vi "Sound sample.vi"() -> ()   [LabVIEW 2016]
uses:
  <vilib>/sound2/lvsound2.llb/Sound Data Format.ctl
  <vilib>/sound2/lvsound2.llb/Sound File Info (path).vi
panel:
  out "sound format":T1={"sample rate (S/s)"=22050.0, "number of channels"=2, "bits per sample"=16}
  out "Waveform Graph":waveform(dbl)(graph)
  in  "Sound  Input":path=path "C:/Users/exception/Desktop/MISC/Public Enemy - Harder Than You Think (HQ).mp3"
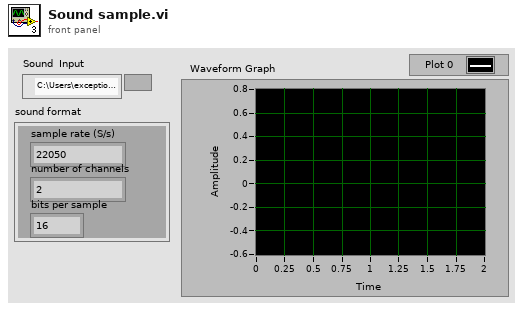
[diagram p1: front panel]
types:
  T1 = typedef "Sound Data Format.ctl" = cluster{"sample rate (S/s)":dbl, "number of channels":i32, "bits per sample":i32}
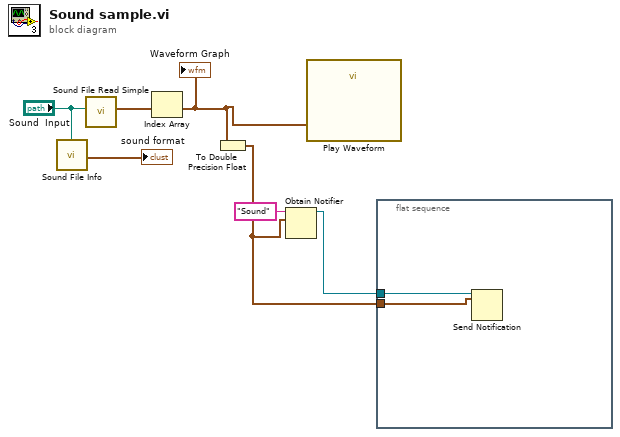
[diagram p0: block diagram]
diagram:
  n1 = call-poly <vilib>:"Sound File Info.vi"("path"="Sound  Input") -> ("sound format"=→"sound format":T1)  [unwired: 7 in, 3 out]
  n2 = call <vilib>:"Sound File Read Simple.vi"("path"="Sound  Input") -> ("data"=w5:waveform(dbl)[])  [unwired: 7 in, 3 out]
  n3 = Index Array(array=w5) -> (element=w2:waveform(dbl))  [unwired: 1 in]
  "Waveform Graph" <- w2
  n4 = To Double Precision Float(number=w2) -> (double precision float=w1:waveform(dbl))
  n5 = Obtain Notifier(name (unnamed)="Sound", notification data type=w1) -> (notifier out=w4:refnum<notifier>)  [unwired: 2 in, 2 out]
  n6 = call "Play Waveform"("Data"=w2) -> ()  [unwired: 18 in, 1 out]
  n7 = flat-sequence {
    tunnel: w4 -> [w9]
    tunnel: w1 -> [w8]
    frame #0 {
      n8 = Send Notification(notification=w8, notifier=w9) -> ()  [unwired: 1 in, 2 out]
    }
  }
